vi "运维调试_总磷总氮.vi"() -> ()   [LabVIEW 2016, in "斯坦道氨氮.lvlib"]
uses:
  <vilib>/Utility/miscctls.llb/LVPointTypeDef.ctl
  <vilib>/Plasmionique/MB Master/MB_Master/MB_Master.lvclass
  <vilib>/ptbypt/NI_PtbyPt.lvlib
panel:
  out "步骤":u16
  out "seconds since 1Jan1904 2":timestamp
  out "seconds since 1Jan1904":timestamp
  in  "周期设置":bool
  in  "流程操作":bool
  out "消解压力":sgl format="%#.2f kPa"
  out "权限等级":string
  out "总步数":i32
  out "滑动杆":dbl(slide) caption="测试进度" scale=0.0..100.0
  out "试剂余量显示":sgl[][](graph)
  in  "仪器校准":bool
  in  "参数查询":bool
  out "简易步骤名称":string
  in  "温度曲线":bool
  in  "试剂余量":bool
  in  "灯值调整":bool
  out "固件版本号":string
  out "模块版本号":string
  out "注射器温度":sgl format="%#.2f ℃"
  out "消解温度":sgl format="%#.2f ℃"
  out "ADC":sgl
  out "F3":sgl format="%#.6f"
  out "F2":sgl format="%#.6f"
  out "F1":sgl format="%#.6f"
  out "F0":sgl format="%#.6f"
  out "运行状态":T1 {"数据时间:" format="%<%y/%m/%d %H:%M:%S>T"; "仪器时间:" format="%<%y/%m/%d %H:%M:%S>T"}
  in  "单选按钮":T2=enum."总氮"
  in  "布尔":bool
  in  "外设固件":bool
  out "字符串 2":string
  in  "数组":string[](array[string])
  in  "返回":bool
  in  "参数设置":bool
  out "集成报警信息":string
  in  "停止":bool
  in  "手动启动":bool
  in  "调试":bool
  out "多列列表框":i32(listbox)
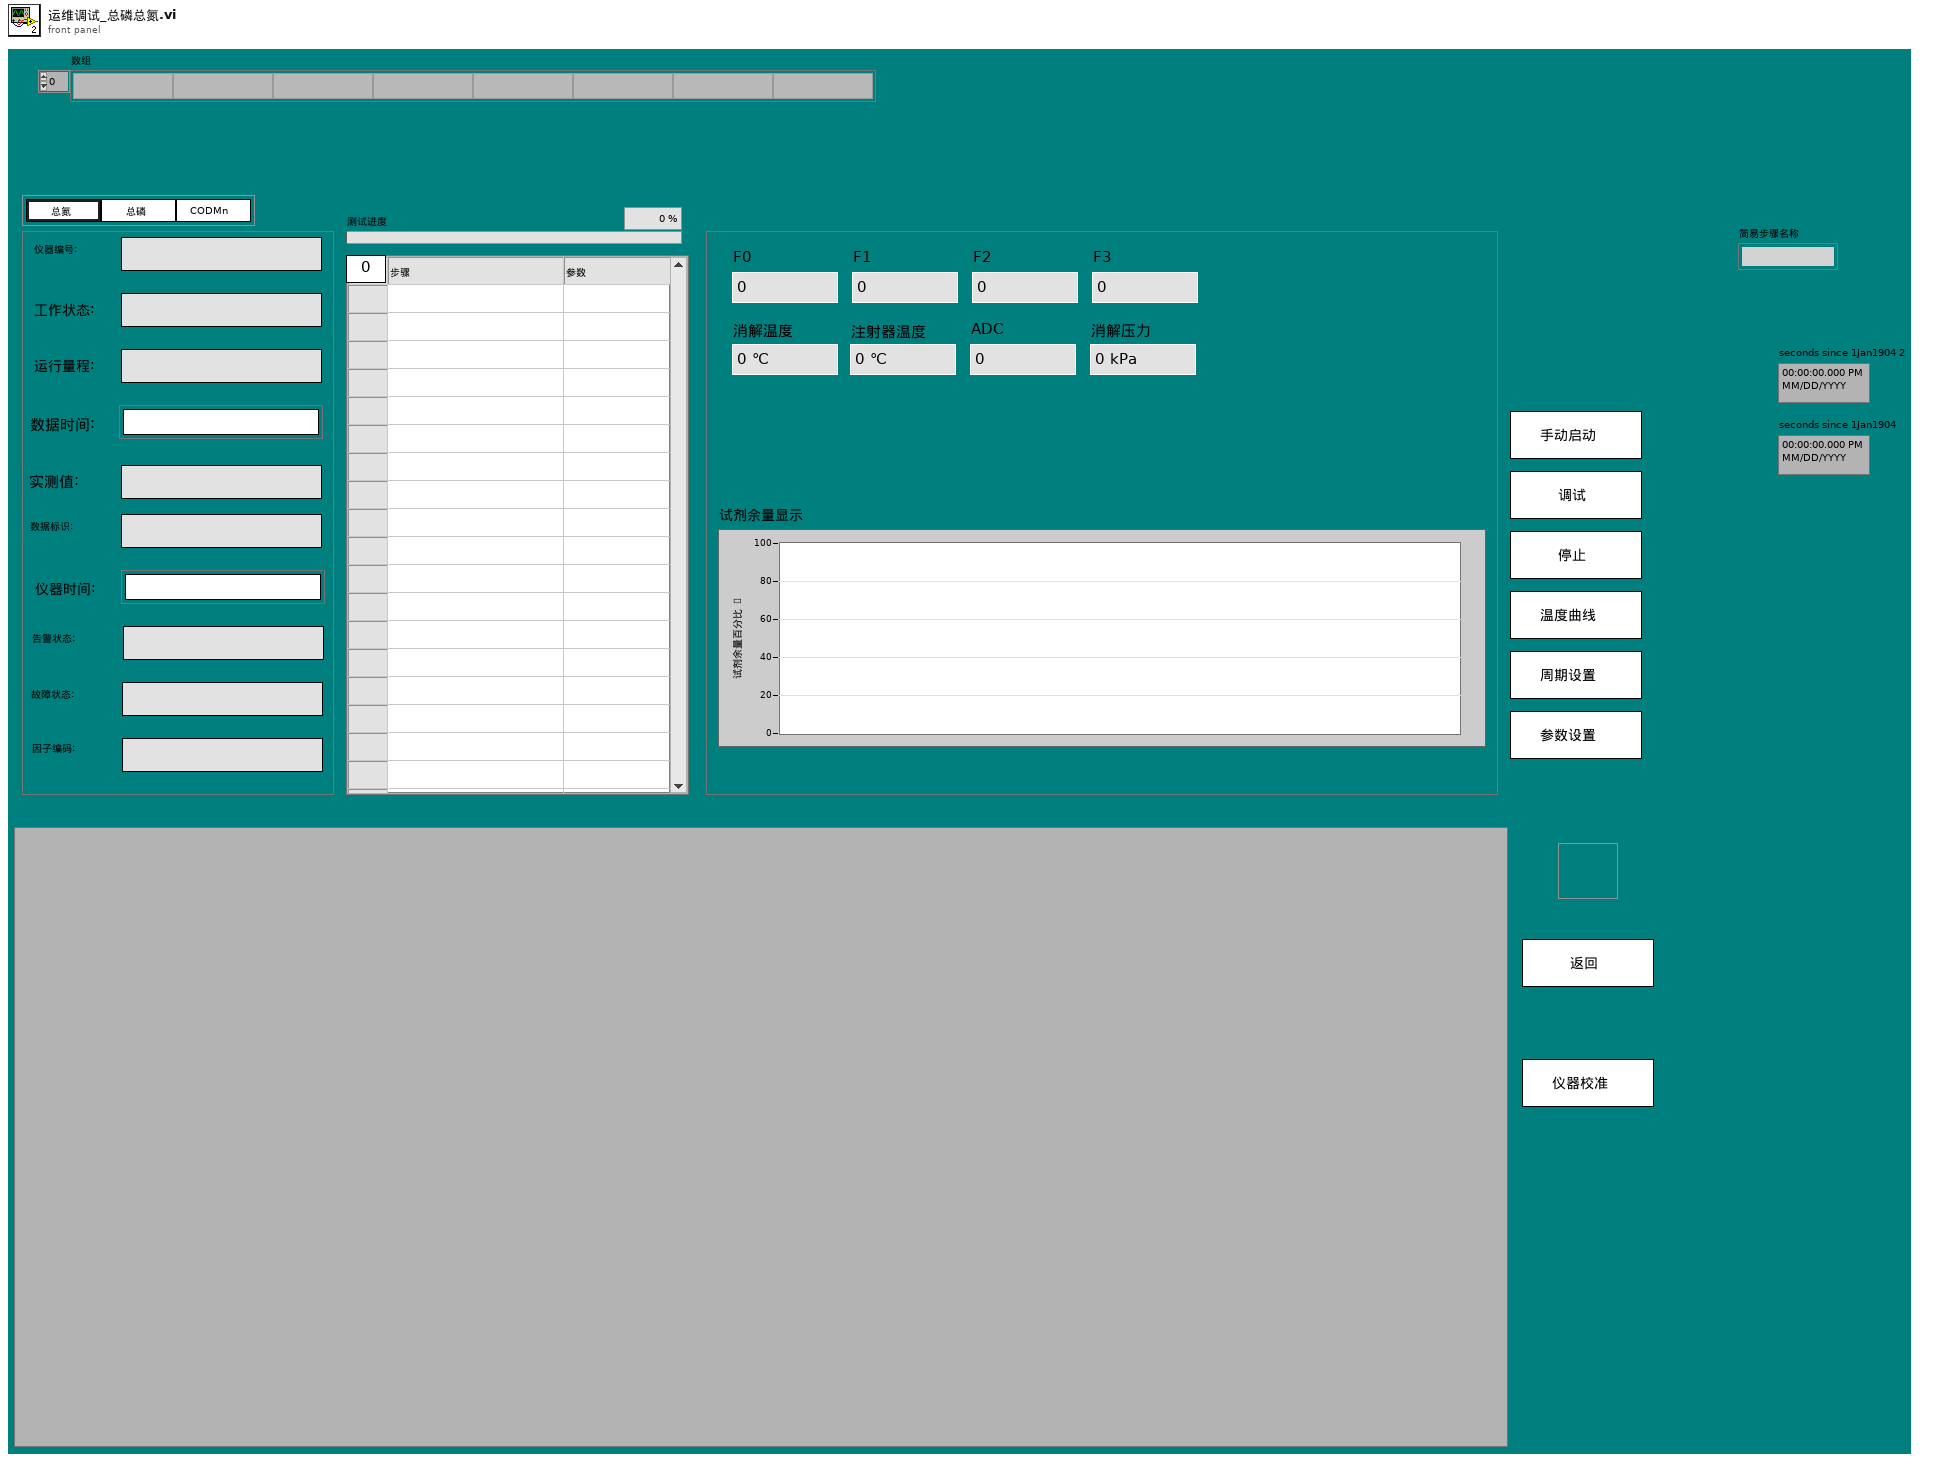
[diagram p1: front panel]
types:
  T1 = cluster{"仪器编号:":string, "工作状态:":string, "运行量程: ":string, "数据时间:":timestamp, "实测值:":string, "数据标识: ":string, "仪器时间:":timestamp, "告警状态: ":string, "故障状态:  ":string, "因子编码:":string}
  T2 = typedef "斯坦道氨氮.lvlib/启动参数显示控件.ctl" = enum32{"COD", "氨氮", "总氮", "总磷", "磷酸盐", "硝氮", "亚硝氮", "硅酸盐", "硫化物", "氟化物", "CODMn"}
  T3 = typedef "LVPointTypeDef.ctl" = cluster{"Horizontal":i16, "Vertical":i16}
  T4 = cluster{"系统时间":timestamp, "工作状态":u16, "测量模式":enum16{"待机", "连续模式", "周期模式", "定点模式", "受控模式", "手动模式"}, "告警代码":u16, "故障代码":u16, "日志代码":u16, "软件版本":u16, "F0":sgl, "F1":sgl, "F2":sgl, "F3":sgl, "T":sgl, "H":sgl, "id":u16, "flowid":u16, "量程":u16, "总磷控温温度1":sgl, "营养盐控温温度2":sgl, "ADC":sgl, "结果值":sgl, "运行时间":u16, "步骤详情":string, "步骤流程":string}
  T5 = typedef "报警信息字段定义.ctl" = cluster{"时间":timestamp, "参数":string, "元器件":string, "故障现象":string, "故障分析":string, "state":string, "code":string, "platform_alarm_code":string, "是否上报":string}
  T6 = typedef "Alarm interface.lvlib/报警短信语音交互.ctl" = cluster{"参数":string, "元器件":string, "故障现象":string, "code":string, "platform_alarm_code":string, "solutionList":cluster{"reason":string, "solution":string}[], "是否上报":string}
  T7 = cluster{"Major":u16, "Minor":u16, "Fix":u16, "Build":u16}
  T8 = typedef "LVStringsAndValuesArrayTypeDef_U16.ctl" = cluster{"String":string, "Value":u16}[]
  T9 = cluster{"因子编码":u32, "单位":u16, "标样参考值":sgl, "水样数据时间":timestamp, "水样实测值":sgl, "水样数据标识":string, "标样数据时间":timestamp, "标样实测值":sgl, "标样数据标识":string, "空白数据时间":timestamp, "空白实测值":sgl, "空白数据标识":string, "零点核查数据时间":timestamp, "零点核查实测值":sgl, "零点核查数据标识":string, "跨度核查数据时间":timestamp, "跨度核查实测值":sgl, "跨度核查数据标识":string, "加标回收数据时间":timestamp, "加标回收实测值":sgl, "加标回收数据标识":string, "平行样数据时间":timestamp, "平行样实测值":sgl, "平行样数据标识":string, "F0":sgl, "F1":sgl, "F2":sgl, "F3":sgl, "F4":sgl, "F5":sgl, "F6":sgl, "F7":sgl, "温度":sgl, "湿度":sgl, "X值":sgl, "fidrange":u16, "X1值":sgl}[]
  T10 = typedef "SingleStepTestV3.lvlib/SingleStepTestV3.lvclass/仪器版本.ctl" = enum16{"V3.1版", "V4版", "V3版", "V4.2版"}
  T11 = cluster{"因子编码":u32, "单位":u16, "标样参考值":sgl, "水样数据时间":timestamp, "水样实测值":sgl, "水样数据标识":string, "标样数据时间":timestamp, "标样实测值":sgl, "标样数据标识":string, "空白数据时间":timestamp, "空白实测值":sgl, "空白数据标识":string, "零点核查数据时间":timestamp, "零点核查实测值":sgl, "零点核查数据标识":string, "跨度核查数据时间":timestamp, "跨度核查实测值":sgl, "跨度核查数据标识":string, "加标回收数据时间":timestamp, "加标回收实测值":sgl, "加标回收数据标识":string, "平行样数据时间":timestamp, "平行样实测值":sgl, "平行样数据标识":string, "F0":sgl, "F1":sgl, "F2":sgl, "F3":sgl, "F4":sgl, "F5":sgl, "F6":sgl, "F7":sgl, "温度":sgl, "湿度":sgl, "X值":sgl, "fidrange":u16, "X1值":sgl}
  T12 = typedef "TimingControl.lvlib/TimingControl.lvclass/国标控制命令.ctl" = enum16{"启动测量", "标样核查", "零点核查", "跨度核查", "空白测试", "平行样测试", "加标回收", "空白校准", "标样校准", "初始化（清洗）", "停止测试", "仪器重启", "校时", "模式设置", "测量间隔设置"}
  T13 = typedef "TimingControl.lvlib/TimingControl.lvclass/测量参数.ctl" = u16
  T14 = enum32{"Bad", "Idle", "Run top level", "Running"}
  T15 = cluster{"时间标识":timestamp, "设备":string, "日志信息":string, "流程参数":string}
  T16 = typedef "LVRowAndColumnUnsignedTypeDef.ctl" = cluster{"Row":u32, "Column":u32}
  T17 = typedef "操作日志字段定义.ctl" = cluster{"时间":timestamp, "参数":string, "日志信息":string, "流程参数":string}
  T18 = cluster{"站号":u16, "量程切换":enum32{"H", "L", "AUTO"}, "控制命令":enum16{"启动测量", "标样核查", "零点核查", "跨度核查", "空白测试", "平行样测试", "加标回收", "空白校准", "标样校准", "初始化（清洗）", "停止测试", "仪器重启", "校时", "模式设置", "测量间隔设置"}, "模式设置":enum16{"待机", "连续模式", "周期模式", "定点模式", "受控模式", "手动模式"}, "测量间隔":u16}
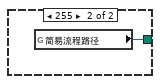
[diagram p6: hidden frame]
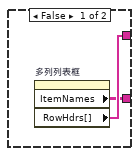
[diagram p7: hidden frame]
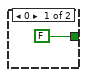
[diagram p11: hidden frame]
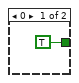
[diagram p18: hidden frame]
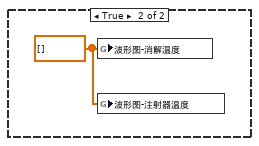
[diagram p19: hidden frame]
diagram:
  n1 = Obtain Queue(name (unnamed)="balloon" ("名称（未命名）"), element data type=cluster{"Title":string, "Body":string} {"Title"="", "Body"=""}) -> (queue out=w1:refnum<queue>)  [unwired: 3 in, 2 out]
  n2 = flat-sequence {
    frame #0 {
      n3 = property on="窗格" class="Pane"("Origin"=T3 {"Horizontal"=0, "Vertical"=0} ("原点")) -> ()  [unwired: 2 in, 2 out]
    }
  }
  n4 = while {
    stop <- FALSE stop-if-true
    n5 = global read "VAR总磷总氮全局变量.vi" "状态告警区"() -> (w32:T4)
    n6 = Wait (ms)(milliseconds to wait=u32 1000 ("等待时间（毫秒）")) -> ()  [unwired: 1 out]
    n7 = Unbundle By Name(w32) -> ("工作状态"=w30:u16)
    n8 = global read "VAR总磷总氮全局变量.vi" "通讯状态"() -> (w33:bool)
    n9 = Equal To 0?(x=w30) -> (x = 0?=w29:bool)
    n10 = And(x=w29, y=w33) -> (x .and. y?=w31:bool)
    n11 = call <vilib>:"Boolean Crossing PtByPt.vi"("input"=w31) -> ("crossing"=w28:bool)  [unwired: 2 in]
    n12 = case shown="True" w28 {
      frame False {
      }
      frame True {
        n13 = control-ref of="试剂余量显示"() -> (w36:refnum<vi>)
        n14 = call "试剂余量展示.vi"("波形图 2"=w36) -> ("波形图"=→"试剂余量显示":sgl[][])  [unwired: 10 in]
      }
    }
  }
  n15 = while {
    shift-right: [w39] -> _
    shift-left: _ -> [w41]
    tunnel: w1 -> [w38]
    stop <- FALSE stop-if-true
    n16 = global read "VAR总磷总氮全局变量.vi" "状态告警区"() -> (w47:T4)
    n17 = Wait (ms)(milliseconds to wait=u32 100 ("等待时间（毫秒）")) -> ()  [unwired: 1 out]
    n18 = Unbundle By Name(w47) -> ("工作状态"=w46:u16, "id"=w45:u16, "日志代码"=w44:u16, "故障代码"=w43:u16, "告警代码"=w42:u16)
    n19 = case shown="1, Default" w46 {
      tunnel: w45 -> [_ w51]
      tunnel: w44 -> [_ w54]
      tunnel: w43 -> [_ w53]
      tunnel: w42 -> [_ w52]
      tunnel: w41 -> [w49 w57]
      tunnel: [w49 w55] -> w39
      tunnel: w38 -> [_ w50]
      frame 0 {
      }
      frame 1, Default {
        n20 = Add(x=w53, y=w52) -> (x+y=w55:u16)
        n21 = Not Equal To 0?(x=w55) -> (x != 0?=w59:bool)
        n22 = Not Equal?(x=w55, y=w57) -> (x != y?=w58:bool)
        n23 = And(x=w59, y=w58) -> (x .and. y?=w56:bool)
        n24 = case shown="True" w56 {
          tunnel: w54 -> [_ _]
          tunnel: w53 -> [_ w64]
          tunnel: w52 -> [_ w63]
          tunnel: w51 -> [_ w60]
          tunnel: w50 -> [_ w68]
          frame False {
          }
          frame True {
            n25 = Not Equal To 0?(x=w64) -> (x != 0?=w66:bool)
            n26 = Not Equal To 0?(x=w63) -> (x != 0?=w62:bool)
            n27 = call "故障码字段定义.vi"("id"=w60, "故障代码"=w64) -> ("告警信息"=w65:T6)  [unwired: 9 in]
            n28 = call "告警码字段定义.vi"("id"=w60, "告警代码"=w63) -> ("告警信息"=w61:T6)  [unwired: 9 in]
            n29 = case shown="True" w66 {
              tunnel: w65 -> [_ w88]
              frame False {
              }
              frame True {
                n30 = Unbundle By Name(w88) -> ("参数"=w87:string, "元器件"=w86:string, "故障现象"=w85:string, "code"=w84:string, "platform_alarm_code"=w83:string, "是否上报"=w82:string)
                n31 = Get Date/Time In Seconds() -> (seconds since 1Jan1904=w89:timestamp)
                n32 = Bundle By Name(cluster=T5 {"时间"=timestamp(0 s since 1904-01-01), "参数"="", "元器件"="", "故障现象"="", "故障分析"="", "state"="", "code"="", "platform_alarm_code"="", "是否上报"=""} ("data in"), "时间"=w89, "参数"=w87, "元器件"=w86, "故障现象"=w85, "code"=w84, "platform_alarm_code"=w83, "是否上报"=w82) -> (w81:T5)
                n33 = call "总磷总氮报警信息.vi"("data in"=w81) -> ()  [unwired: 10 in, 1 out]
              }
            }
            n34 = Unbundle By Name(w65) -> ("故障现象"=w70:string)
            n35 = Unbundle By Name(w61) -> ("故障现象"=w69:string)
            n36 = case shown="True" w62 {
              tunnel: w61 -> [_ w71]
              frame False {
              }
              frame True {
                n37 = Unbundle By Name(w71) -> ("参数"=w75:string, "元器件"=w76:string, "故障现象"=w77:string, "code"=w78:string, "platform_alarm_code"=w79:string, "是否上报"=w80:string)
                n38 = Get Date/Time In Seconds() -> (seconds since 1Jan1904=w74:timestamp)
                n39 = Bundle By Name(cluster=T5 {"时间"=timestamp(0 s since 1904-01-01), "参数"="", "元器件"="", "故障现象"="", "故障分析"="", "state"="", "code"="", "platform_alarm_code"="", "是否上报"=""} ("data in"), "时间"=w74, "参数"=w75, "元器件"=w76, "故障现象"=w77, "code"=w78, "platform_alarm_code"=w79, "是否上报"=w80) -> (w72:T5)
                n40 = call "总磷总氮报警信息.vi"("data in"=w72) -> ()  [unwired: 10 in, 1 out]
              }
            }
            n41 = Bundle("故障现象"=w70, "故障现象"=w69) -> (w67:cluster{"故障现象":string, "故障现象":string})  [unwired: 1 in]
            n42 = Enqueue Element(queue=w68, element=w67) -> ()  [unwired: 2 in, 3 out]
          }
        }
      }
    }
  }
  n43 = flat-sequence {
    tunnel: [w137] -> w20
    tunnel: [errorcluster {"status"=FALSE, "code"=0, "source"=""} ("错误输入（无错误）")] -> w11
    tunnel: [errorcluster {"status"=FALSE, "code"=0, "source"=""} ("错误输入（无错误）")] -> w10
    tunnel: [w134] -> w8
    tunnel: [errorcluster {"status"=FALSE, "code"=0, "source"=""} ("error out")] -> w7
    tunnel: [errorcluster {"status"=FALSE, "code"=0, "source"=""} ("错误输入（无错误）")] -> w6
    frame #0 {
      n44 = global read "VAR总磷总氮全局变量.vi" "初始化"() -> (w91:bool)
      n45 = control-ref of="本VI"() -> (w99:refnum<vi>)
      n46 = case shown="False" w91 {
        frame False {
          n47 = call "配置初始化.vi"() -> ()  [unwired: 11 in, 1 out]
        }
        frame True {
        }
      }
      n48 = property class="VI"(reference=w99) -> ("Library.Version"=w98:T7)  [unwired: 1 in, 2 out]
      n49 = Unbundle By Name(w98) -> ("Major"=w96:u16, "Minor"=w95:u16, "Fix"=w94:u16, "Build"=w93:u16)
      n50 = Format Into String(format string="模块版本号：%d.%d.%d.%d" ("格式字符串"), w96, w95, w94, w93) -> (resulting string=→"模块版本号":string)  [unwired: 2 in, 1 out]
      n51 = call "新建通讯互斥锁.vi"() -> ()  [unwired: 11 in, 1 out]
    }
    frame #1 {
      n52 = vi-ref "斯坦道氨氮.lvlib:总磷总氮通讯.vi"() -> (w104:refnum<vi>)
      n53 = global read "model config var.vi" "启动队列名称"() -> (w102:cluster{"String":string, "Value":u16}[])
      n54 = vi-ref "斯坦道氨氮.lvlib:总磷总氮测量数据储存.vi"() -> (w112:refnum<vi>)
      n55 = property class="VI"(reference=w104) -> ("Name"=w105:string)  [unwired: 1 in, 2 out]
      n56 = Index Array(array=w102) -> (element=w101:cluster{"String":string, "Value":u16})  [unwired: 1 in]
      n57 = Unbundle By Name(w101) -> ("Value"=w100:u16)
      n58 = property class="VI"(reference=w112) -> ("Name"=w119:string)  [unwired: 1 in, 2 out]
      n59 = Open VI Reference(type specifier VI Refnum (for type only)=refnum<vi> refnum, vi path=w105, options=128 ("选项")) -> (vi reference=w107:refnum<vi>, error out=w109:errorcluster)  [unwired: 3 in]
      n60 = case shown="22" w100 {
        tunnel: [w120 启动参数显示控件."总磷" ("单选按钮") 启动参数显示控件."总氮" ("单选按钮") 启动参数显示控件."COD" ("单选按钮") 启动参数显示控件."氨氮" ("单选按钮") 启动参数显示控件."磷酸盐" ("单选按钮") 启动参数显示控件."硝氮" ("单选按钮") 启动参数显示控件."亚硝氮" ("单选按钮") 启动参数显示控件."硅酸盐" ("单选按钮") 启动参数显示控件."硫化物" ("单选按钮") 启动参数显示控件."氟化物" ("单选按钮") 启动参数显示控件."CODMn" ("单选按钮")] -> w103
        frame 0, Default {
          n61 = property on="单选按钮" class="RadioBtnsControl (strict)"() -> ("Value"=w120:T2)  [unwired: 2 in, 2 out]
        }
        frame 1 {
        }
        frame 2 {
        }
        frame 22 {
        }
        frame 3 {
        }
        frame 4 {
        }
        frame 5 {
        }
        frame 6 {
        }
        frame 7 {
        }
        frame 8 {
        }
        frame 50 {
        }
        frame 21 {
        }
      }
      n62 = call-by-ref "开始异步调用"(reference=w107, error in=w109) -> (reference out=w111:refnum<vi>, error out=w110:errorcluster)  [unwired: 12 in]
      n63 = Open VI Reference(type specifier VI Refnum (for type only)=refnum<vi> refnum, vi path=w119, options=128 ("选项")) -> (vi reference=w117:refnum<vi>, error out=w115:errorcluster)  [unwired: 3 in]
      n64 = Close Reference(reference=w111, error in (no error)=w110) -> ()  [unwired: 1 out]
      n65 = call-by-ref "开始异步调用"(reference=w117, error in=w115) -> (reference out=w113:refnum<vi>, error out=w114:errorcluster)  [unwired: 12 in]
      n66 = Close Reference(reference=w113, error in (no error)=w114) -> ()  [unwired: 1 out]
      n67 = property on="单选按钮" class="RadioBtnsControl (strict)"("Value"=w103) -> ()  [unwired: 2 in, 2 out]
    }
    frame #2 {
      n68 = call "配置文件路径.vi"() -> ("appended path"=w134:path)  [unwired: 11 in]
      n69 = call "设置模块队列名.vi"() -> ("Msg"=w137:string)  [unwired: 5 in]
    }
  }
  n70 = while {
    shift-right: [w147] -> _
    shift-left: u32 0 ("y") -> [w149]
    stop <- FALSE stop-if-true
    # "密码权限"
    n71 = global read "VAR总磷总氮全局变量.vi" "权限等级"() -> (w144:enum16{"一级权限", "二级权限", "三级权限", "超级权限"})
    n72 = case shown="False" "布尔" {
      tunnel: w149 -> [_ w162]
      tunnel: [_ w161] -> w147
      frame False {
      }
      frame True {
        n73 = Increment(x=w162) -> (x+1=w161:u32)
      }
    }
    n74 = Wait (ms)(milliseconds to wait=u32 1000 ("等待时间（毫秒）")) -> ()  [unwired: 1 out]
    n75 = case shown="\"超级权限\"" w144 {
      tunnel: [_ w154 w156 w159] -> w138
      tunnel: [_ _ w156 w159] -> _
      tunnel: [_ w154 w156 w159] -> w143
      tunnel: [_ _ _ TRUE] -> _
      tunnel: [TRUE _ _ _] -> w141
      tunnel: ["一级权限" "二级权限" "三级权限" "超级权限"] -> w139
      frame "一级权限", Default {
      }
      frame "二级权限" {
        w154 = TRUE
      }
      frame "三级权限" {
        w156 = TRUE
      }
      frame "超级权限" {
        w159 = TRUE
      }
    }
    "权限等级" <- w139
    n76 = property on="外设固件" class="Bool"("Visible"=w143) -> ()  [unwired: 2 in, 2 out]
    n77 = property on="流程操作" class="Bool"("Visible"=w138) -> ()  [unwired: 2 in, 2 out]
    n78 = property on="试剂余量" class="Bool"("Visible"=w138) -> ()  [unwired: 2 in, 2 out]
    n79 = property on="灯值调整" class="Bool"("Visible"=w138) -> ()  [unwired: 2 in, 2 out]
    n80 = Greater Or Equal?(x=w147, y=u32 3600) -> (x >= y?=w145:bool)
    n81 = Not(x=w141) -> (.not. x?=w140:bool)
    n82 = property on="布尔" class="Bool (strict)"("Value"=w140) -> ()  [unwired: 2 in, 2 out]
    n83 = case shown="True" w145 {
      frame False {
      }
      frame True {
        n84 = global write "VAR总磷总氮全局变量.vi" "权限等级"(enum16{"一级权限", "二级权限", "三级权限", "超级权限"}."一级权限" ("权限等级")) -> ()
      }
    }
  }
  n85 = while {
    shift-right: [w167] -> _
    shift-left: 0 -> [w168]
    stop <- FALSE stop-if-true
    n86 = global read "VAR总磷总氮全局变量.vi" "心跳包打开状态"() -> (w163:bool)
    n87 = Wait (ms)(milliseconds to wait=u32 1000 ("等待时间（毫秒）")) -> ()  [unwired: 1 out]
    n88 = case shown="False" w163 {
      tunnel: w168 -> [w172 _]
      tunnel: [w171 _] -> w167
      frame False {
        n89 = Increment(x=w172) -> (x+1=w171:i32)
      }
      frame True {
      }
    }
    n90 = Greater Or Equal?(x=w167, y=600) -> (x >= y?=w165:bool)
    n91 = case shown="True" w165 {
      frame False {
      }
      frame True {
        n92 = global write "VAR总磷总氮全局变量.vi" "升级固件关闭心跳包"(FALSE ("关闭心跳包")) -> ()
      }
    }
  }
  n93 = while {
    shift-right: [w174] -> _
    shift-left: TRUE -> [w175]
    stop <- FALSE stop-if-true
    n94 = global read "VAR总磷总氮全局变量.vi" "状态告警区"() -> (w178:T4)
    n95 = global read "VAR总磷总氮全局变量.vi" "状态告警区"() -> (w181:T4)
    n96 = Wait (ms)(milliseconds to wait=u32 1000 ("等待时间（毫秒）")) -> ()  [unwired: 1 out]
    n97 = Unbundle By Name(w181) -> ("工作状态"=w176:u16, "总磷控温温度1"=w180:sgl, "营养盐控温温度2"=w179:sgl)
    n98 = Unbundle By Name(w178) -> ("总磷控温温度1"=w177:sgl)
    n99 = call "消解压力计算.vi"("当前消解温度"=w177) -> ("消解压力"=→"消解压力":dbl)  [unwired: 10 in]
    n100 = case shown="1, Default" w176 {
      tunnel: w180 -> [_ w187]
      tunnel: w179 -> [_ w186]
      tunnel: w175 -> [_ w185]
      tunnel: [TRUE _] -> w174
      frame 0 {
      }
      frame 1, Default {
        n101 = case shown="False" w185 {
          tunnel: w187 -> [w193 _]
          tunnel: w186 -> [w192 _]
          frame False {
            n102 = global read "VAR总磷总氮全局变量.vi" "波形图-消解温度"() -> (w191:sgl[])
            n103 = global read "VAR总磷总氮全局变量.vi" "波形图-注射器温度"() -> (w190:sgl[])
            n104 = Build Array (concatenate)(w191, w193) -> (w189:sgl[])
            n105 = Build Array (concatenate)(w190, w192) -> (w188:sgl[])
            n106 = global write "VAR总磷总氮全局变量.vi" "波形图-消解温度"(w189) -> ()
            n107 = global write "VAR总磷总氮全局变量.vi" "波形图-注射器温度"(w188) -> ()
          }
          frame True {
            w194 = dbl[] [] ("波形图-消解温度")
            n108 = global write "VAR总磷总氮全局变量.vi" "波形图-消解温度"(w194) -> ()
            n109 = global write "VAR总磷总氮全局变量.vi" "波形图-注射器温度"(w194) -> ()
          }
        }
      }
    }
  }
  n110 = while {
    stop <- FALSE stop-if-true
    n111 = global read "VAR总磷总氮全局变量.vi" "状态告警区"() -> (w206:T4)
    n112 = Wait (ms)(milliseconds to wait=u32 1000 ("等待时间（毫秒）")) -> ()  [unwired: 1 out]
    n113 = Unbundle By Name(w206) -> ("id"=w205:u16, "flowid"=w204:u16, "量程"=w203:u16, "工作状态"=w196:u16)
    n114 = case shown="0, Default" w196 {
      tunnel: [w216 w217] -> w198
      frame 0, Default {
        n115 = global read "总磷总氮断电保存全局变量.vi" "流程路径"() -> (w216:path)
      }
      frame 255 {
        n116 = global read "总磷总氮断电保存全局变量.vi" "简易流程路径"() -> (w217:path)
      }
    }
    n117 = feedback #1() -> (w195:u16)  [unwired: 1 in]
    n118 = feedback-in #1(w196) -> ()
    n119 = Not Equal?(x=w195, y=w196) -> (x != y?=w212:bool)
    n120 = Not Equal To 0?(x=w196) -> (x != 0?=w207:bool)
    n121 = Bundle("id"=w205, "flowid"=w204, "量程"=w203) -> (w200:cluster{"id":u16, "flowid":u16, "量程":u16})  [unwired: 1 in]
    n122 = feedback #2() -> (w197:path)  [unwired: 1 in]
    n123 = feedback-in #2(w198) -> ()
    n124 = feedback-in #3(w200) -> ()
    n125 = feedback #3() -> (w201:cluster{"id":u16, "flowid":u16, "量程":u16})  [unwired: 1 in]
    n126 = Not Equal?(x=w197, y=w198) -> (x != y?=w211:bool)
    n127 = Not Equal?(x=w200, y=w201) -> (x != y?=w199:bool)
    n128 = Compound Arithmetic op=OR ("复合运算")(w211, w212, w199) -> (w213:bool)
    n129 = And(x=w207, y=w213) -> (x .and. y?=w208:bool)
    n130 = case shown="True" w208 {
      tunnel: [w219 w222] -> w210
      tunnel: [w218 w223] -> w214
      tunnel: w200 -> [_ w221]
      tunnel: w198 -> [_ w224]
      tunnel: w196 -> [_ w220]
      frame False {
        n131 = property on="多列列表框" class="MCListbox (strict)"() -> ("ItemNames"=w218:string[][], "RowHdrs[]"=w219:string[])  [unwired: 2 in, 2 out]
      }
      frame True {
        n132 = case shown="255" w220 {
          tunnel: w221 -> [_ w229]
          frame 0, Default {
          }
          frame 255 {
            n133 = Unbundle By Name(w229) -> ("id"=w228:u16, "flowid"=w226:u16)
            n134 = call "获取简易流程名称API.vi"("参数下拉列表"=w228) -> ("字符串与值[]"=w227:T8)  [unwired: 9 in, 1 out]
            n135 = for {
              tunnel: w227 -> [w234] mode=indexing
              tunnel: w226 -> [w232]
              tunnel: [w231] -> w225
              stop <- w230 stop-if-true
              n136 = Unbundle By Name(w234) -> ("String"=w231:string, "Value"=w233:u16)
              n137 = Equal?(x=w233, y=w232) -> (x = y?=w230:bool)
            }
            "简易步骤名称" <- w225
          }
        }
        n138 = call "斯坦道XML解析.vi"("工作状态"=w220, "添加的路径"=w224, "参数簇"=w221) -> ("步骤名"=w223:string[][], "索引"=w222:string[])  [unwired: 6 in, 1 out]
      }
    }
    n139 = Array Size(array=w210) -> (size(s)=→"总步数":i32)
    n140 = property on="多列列表框" class="MCListbox (strict)"("ItemNames"=w214, "RowHdrs[]"=w210) -> ()  [unwired: 2 in, 2 out]
  }
  n141 = while {
    shift-right: [w246] -> _
    shift-left: u16 1 ("工作状态") -> [w244]
    stop <- FALSE stop-if-true
    (unwired) "注射器温度"
    n142 = global write "VAR总磷总氮全局变量.vi" "最近一次工作状态"(w244) -> ()
    n143 = global read "VAR总磷总氮全局变量.vi" "状态告警区"() -> (w266:T4)
    n144 = global read "VAR总磷总氮全局变量.vi" "通讯状态"() -> (w277:bool)
    n145 = Wait (ms)(milliseconds to wait=u32 1000 ("等待时间（毫秒）")) -> ()  [unwired: 1 out]
    n146 = case shown="\"氨氮\"" "单选按钮" {
      tunnel: [22 3 2 1 4 5 6 7 8 50 21] -> w235
      tunnel: [_ TRUE _ _ _ _ _ _ _ _ _] -> w238
      frame "COD", Default {
      }
      frame "氨氮" {
      }
      frame "总氮" {
      }
      frame "总磷" {
      }
      frame "磷酸盐" {
      }
      frame "硝氮" {
      }
      frame "亚硝氮" {
      }
      frame "硅酸盐" {
      }
      frame "硫化物" {
      }
      frame "氟化物" {
      }
      frame "CODMn" {
      }
    }
    n147 = Unbundle By Name(w266) -> ("id"=w265:u16, "工作状态"=w261:u16)
    n148 = case shown="True" w277 {
      tunnel: ["通讯异常" ("集成报警信息") w396] -> w276
      frame False {
      }
      frame True {
        n149 = local read "seconds since 1Jan1904 2"() -> (w388:timestamp)
        n150 = local read "seconds since 1Jan1904"() -> (w391:timestamp)
        n151 = global read "VAR总磷总氮全局变量.vi" "状态告警区"() -> (w398:T4)
        n152 = Unbundle By Name(w398) -> ("工作状态"=w394:u16)
        n153 = Subtract(x=w388, y=w391) -> (x-y=w387:dbl)
        n154 = Not Equal To 0?(x=w394) -> (x != 0?=w390:bool)
        n155 = Get Date/Time In Seconds() -> (seconds since 1Jan1904=w389:timestamp)
        n156 = case shown="True" w390 {
          tunnel: w389 -> [_ w399]
          frame False {
          }
          frame True {
            "seconds since 1Jan1904 2" <- w399
          }
        }
        n157 = Greater Or Equal?(x=w387, y=36000.0) -> (x >= y?=w384:bool)
        n158 = call <vilib>:"Boolean Crossing PtByPt.vi"("direction"=enum16{"either", "false-true", "true-false"}."false-true", "input"=w390) -> ("crossing"=w392:bool)  [unwired: 1 in]
        n159 = Or(x=w392, y=w384) -> (x .or. y?=w385:bool)
        n160 = case shown="True" w385 {
          tunnel: w389 -> [_ w400]
          frame False {
          }
          frame True {
            "seconds since 1Jan1904" <- w400
          }
        }
        n161 = global read "VAR总磷总氮全局变量.vi" "测量状态"() -> (w395:string)
        n162 = Format Into String(format string="工作计时: %d 秒" ("格式字符串"), initial string=w395, w387) -> (resulting string=w396:string)  [unwired: 1 in, 1 out]
      }
    }
    "集成报警信息" <- w276
    n163 = global read "VAR总磷总氮全局变量.vi" "测量数据区数组"() -> (w250:T9)
    n164 = case shown="1, Default" w261 {
      tunnel: w265 -> [_ w333]
      frame 0 {
      }
      frame 1, Default {
        n165 = case shown="3" w333 {
          tunnel: [w334 启动参数显示控件."总磷" ("单选按钮") 启动参数显示控件."总氮" ("单选按钮") 启动参数显示控件."COD" ("单选按钮") 启动参数显示控件."氨氮" ("单选按钮") 启动参数显示控件."磷酸盐" ("单选按钮") 启动参数显示控件."硝氮" ("单选按钮") 启动参数显示控件."亚硝氮" ("单选按钮") 启动参数显示控件."硅酸盐" ("单选按钮") 启动参数显示控件."硫化物" ("单选按钮") 启动参数显示控件."CODMn" ("单选按钮") 启动参数显示控件."氟化物" ("单选按钮")] -> w332
          frame 0, Default {
            n166 = property on="单选按钮" class="RadioBtnsControl (strict)"() -> ("Value"=w334:T2)  [unwired: 2 in, 2 out]
          }
          frame 1 {
          }
          frame 2 {
          }
          frame 22 {
          }
          frame 3 {
          }
          frame 4 {
          }
          frame 5 {
          }
          frame 6 {
          }
          frame 7 {
          }
          frame 8 {
          }
          frame 21 {
          }
          frame 50 {
          }
        }
        n167 = property on="单选按钮" class="RadioBtnsControl (strict)"("Value"=w332) -> ()  [unwired: 2 in, 2 out]
      }
    }
    n168 = call "版本判断.vi"() -> ("仪器版本"=w240:T10)  [unwired: 11 in]
    n169 = call "id参数转换.vi"("id"=w235) -> ("数组资源索引"=w247:i32)  [unwired: 9 in, 1 out]
    n170 = case shown="\"V4版\", \"V4.2版\"" w240 {
      tunnel: [w280 "传感器" ("标题.文本")] -> w237
      tunnel: ["%#.2f ℃" ("数值文本.格式字符串") "%#.2f " ("数值文本.格式字符串")] -> w239
      tunnel: w238 -> [w283 _]
      frame "V3.1版", Default {
        n171 = Select(t="显色温度", s=w283, f="注射器温度" ("标题.文本")) -> (s? t:f=w280:string)
      }
      frame "V4版", "V4.2版" {
      }
    }
    n172 = Index Array(array=w250, index=w247) -> (element=w249:T11)
    n173 = case shown="0, Default" w244 {
      tunnel: [w301 w307 w311 w315 w319 w323 w327 w331] -> w260
      tunnel: [w299 w306 w310 w314 w317 w322 w326 w330] -> w255
      tunnel: [w302 w305 w309 w313 w316 w321 w325 w329] -> w253
      tunnel: w249 -> [_ w304 w308 w312 w318 w320 w324 w328]
      frame 0, Default {
        n174 = local read "运行状态"() -> (w303:T1)
        n175 = Unbundle By Name(w303) -> ("数据时间:"=w301:timestamp, "实测值:"=w300:string, "数据标识:"=w302:string)
        n176 = Fract/Exp String To Number(string=w300) -> (number=w299:dbl)  [unwired: 3 in, 1 out]
      }
      frame 1 {
        n177 = Unbundle By Name(w304) -> ("水样数据时间"=w307:timestamp, "水样实测值"=w306:sgl, "水样数据标识"=w305:string)
      }
      frame 2, 9 {
        n178 = Unbundle By Name(w308) -> ("标样数据时间"=w311:timestamp, "标样实测值"=w310:sgl, "标样数据标识"=w309:string)
      }
      frame 3 {
        n179 = Unbundle By Name(w312) -> ("零点核查数据时间"=w315:timestamp, "零点核查实测值"=w314:sgl, "零点核查数据标识"=w313:string)
      }
      frame 4 {
        n180 = Unbundle By Name(w318) -> ("跨度核查数据时间"=w319:timestamp, "跨度核查实测值"=w317:sgl, "跨度核查数据标识"=w316:string)
      }
      frame 7 {
        n181 = Unbundle By Name(w320) -> ("加标回收数据时间"=w323:timestamp, "加标回收实测值"=w322:sgl, "加标回收数据标识"=w321:string)
      }
      frame 5, 8 {
        n182 = Unbundle By Name(w324) -> ("空白数据时间"=w327:timestamp, "空白实测值"=w326:sgl, "空白数据标识"=w325:string)
      }
      frame 6 {
        n183 = Unbundle By Name(w328) -> ("平行样数据时间"=w331:timestamp, "平行样实测值"=w330:sgl, "平行样数据标识"=w329:string)
      }
    }
    n184 = Unbundle By Name(w249) -> ("因子编码"=w251:u32)
    n185 = global read "VAR总磷总氮全局变量.vi" "状态告警区"() -> (w275:T4)
    n186 = Unbundle By Name(w275) -> ("flowid"=w243:u16, "系统时间"=w271:timestamp, "工作状态"=w270:u16, "告警代码"=w264:u16, "故障代码"=w263:u16, "量程"=w269:u16)
    n187 = case shown="2" w270 {
      selector: w270 -> [w350 _ w356 w360 w363 w365 w367 w369 w371 w373 w375 w377 w379 w382]
      tunnel: [w351 "空闲" ("工作状态") "水样测量" ("工作状态") w359 "零点核查" ("工作状态") "跨度核查" ("工作状态") "空白测试" ("工作状态") "平行样测试" ("工作状态") "加标回收" ("工作状态") "空白校准" ("工作状态") "标样校准" ("工作状态") "初始化" ("工作状态") "单步调试" ("工作状态") w381] -> w245
      tunnel: [w349 w354 w356 w360 w363 w365 w367 w369 w371 w373 w375 w377 w379 w382] -> w246
      tunnel: w244 -> [w349 w354 _ _ _ _ _ _ _ _ _ _ _ _]
      tunnel: w243 -> [_ _ _ w358 _ _ _ _ _ _ _ _ _ _]
      frame Default {
        n188 = Format Into String(format string="%d" ("格式字符串"), initial string="未知" ("工作状态"), w350) -> (resulting string=w351:string)  [unwired: 1 in, 1 out]
      }
      frame 0 {
      }
      frame 1 {
      }
      frame 2 {
        n189 = case shown="5" w358 {
          tunnel: ["标样核查" ("工作状态") "快捷测试" ("工作状态")] -> w359
          frame 0, Default {
          }
          frame 5 {
          }
        }
      }
      frame 3 {
      }
      frame 4 {
      }
      frame 5 {
      }
      frame 6 {
      }
      frame 7 {
      }
      frame 8 {
      }
      frame 9 {
      }
      frame 10 {
      }
      frame 254 {
      }
      frame 255 {
        n190 = local read "简易步骤名称"() -> (w381:string)
      }
    }
    n191 = call "告警码字段定义.vi"("id"=w235, "告警代码"=w264) -> ("告警信息"=w242:T6)  [unwired: 9 in]
    n192 = call "故障码字段定义.vi"("id"=w235, "故障代码"=w263) -> ("告警信息"=w262:T6)  [unwired: 9 in]
    n193 = Unbundle By Name(w242) -> ("故障现象"=w241:string)
    n194 = Unbundle By Name(w262) -> ("故障现象"=w236:string)
    n195 = property on="注射器温度" class="DigNum (strict)"("Caption.Text"=w237, "NumText.FormatString"=w239) -> ()  [unwired: 2 in, 2 out]
    n196 = case shown="1" w269 {
      tunnel: ["" ("字符串") "低量程 " ("字符串") "高量程 " ("字符串")] -> w268
      frame Default {
      }
      frame 0 {
      }
      frame 1 {
      }
    }
    n197 = Number To Fractional String(number=w255, precision (6)=i16 4 ("精度(6)")) -> (F-format string=w257:string)  [unwired: 2 in]
    n198 = Concatenate Strings(w257, " " ("字符串"), "mg/L" ("字符串")) -> (w254:string)
    n199 = global read "VAR总磷总氮全局变量.vi" "序列号"() -> (w272:string)
    n200 = Format Into String(format string="w%05d" ("格式字符串"), w251) -> (resulting string=w267:string)  [unwired: 2 in, 1 out]
    n201 = global write "VAR总磷总氮全局变量.vi" "工作状态:"(w245) -> ()
    n202 = Bundle By Name(cluster=T1 {"仪器编号:"="", "工作状态:"="", "运行量程: "="", "数据时间:"=timestamp(0 s since 1904-01-01), "实测值:"="", "数据标识: "="", "仪器时间:"=timestamp(0 s since 1904-01-01), "告警状态: "="", "故障状态:  "="", "因子编码:"=""} ("运行状态"), "仪器编号:"=w272, "仪器时间:"=w271, "工作状态:"=w245, "告警状态:"=w241, "故障状态:"=w236, "运行量程:"=w268, "数据时间:"=w260, "实测值:"=w254, "数据标识:"=w253, "因子编码:"=w267) -> (→"运行状态":T1)
  }
  n203 = while {
    shift-right: [w401] -> _
    shift-left: _ -> [w406]
    tunnel: w8 -> [w404]
    stop <- FALSE stop-if-true
    n204 = File/Directory Info(path=w404) -> (last mod=w401:timestamp, error out=w402:errorcluster)  [unwired: 1 in, 5 out]
    n205 = Wait (ms)(milliseconds to wait=u32 1000 ("等待时间（毫秒）")) -> ()  [unwired: 1 out]
    n206 = Not Equal?(x=w406, y=w401) -> (x != y?=w405:bool)
    n207 = case shown="True" w405 {
      tunnel: [_ w408] -> _
      tunnel: w402 -> [_ _]
      frame False {
      }
      frame True {
        n208 = call "配置初始化.vi"() -> ("error out"=w408:errorcluster)  [unwired: 11 in]
      }
    }
  }
  n209 = flat-sequence {
    tunnel: w7 -> [_]
    frame #0 {
      (unwired) u32 0 ("等待时间（毫秒）")
      n210 = control-ref of="周期设置"() -> (w413:refnum<vi>)
      n211 = call "试剂余量后台任务.vi"() -> ()  [unwired: 12 in]
      n212 = call "New TimingControl.vi"("Reference"=w413) -> ("error out"=w411:errorcluster, "TimingControl out"=w412:refnum<class "TimingControl.lvclass">)  [unwired: 9 in]
      n213 = call "taskqueue ref.vi"() -> ("队列输出"=w414:refnum<queue>)  [unwired: 10 in, 1 out]
      n214 = while {
        tunnel: w414 -> [w433]
        shift-right: [w426] -> w410
        shift-left: w412 -> [w431]
        shift-right: [w425] -> w409
        shift-left: w411 -> [w430]
        stop <- FALSE stop-if-true
        n215 = global read "VAR总磷总氮全局变量.vi" "状态告警区"() -> (w434:T4)
        n216 = Wait (ms)(milliseconds to wait=u32 500 ("等待时间（毫秒）")) -> ()  [unwired: 1 out]
        n217 = global read "model config var.vi" "启动队列名称"() -> (w420:cluster{"String":string, "Value":u16}[])
        n218 = Unbundle By Name(w434) -> ("工作状态"=w432:u16, "系统时间"=w428:timestamp)
        n219 = for {
          tunnel: w420 -> [w445] mode=indexing
          tunnel: [w444] -> w419 mode=indexing
          n220 = Unbundle By Name(w445) -> ("String"=w444:string)
        }
        n221 = case shown="1, Default" w432 {
          tunnel: [FALSE TRUE] -> w427
          frame 0 {
          }
          frame 1, Default {
          }
        }
        n222 = property class="TimingControl"(reference=w431, error in=w430, "Properties:仪器时间"=w428, "Properties:仪器运行状态"=w427) -> (reference out=w426:refnum<class "TimingControl.lvclass">, error out=w425:errorcluster, "Properties:命令输出"=w429:cluster{"启动":bool, "控制命令":T12, "测量参数":T13})
        n223 = Array To Spreadsheet String(delimiter (Tab)="/" ("分隔符(Tab)"), array=w419, 3:"" ("格式字符串")) -> (spreadsheet string=w422:string)
        n224 = Unbundle By Name(w429) -> ("启动"=w416:bool, "控制命令"=w418:T12)
        n225 = Insert Into Array(array=w419, new element=w422) -> (w421:string[])  [unwired: 1 in]
        n226 = Bundle(w421) -> ()  [unwired: 1 in, 1 out]
        n227 = Bundle("控制命令"=w418, "") -> (w417:cluster{"控制命令":T12, string})  [unwired: 1 in]
        n228 = case shown="True" w416 {
          tunnel: w417 -> [_ w438]
          tunnel: w433 -> [_ w441]
          frame False {
          }
          frame True {
            n229 = Get Queue Status(queue=w441) -> (queue out=w439:refnum<queue>, # elements in queue=w440:i32)  [unwired: 2 in, 6 out]
            n230 = Equal To 0?(x=w440) -> (x = 0?=w437:bool)
            n231 = case shown="True" w437 {
              tunnel: w439 -> [_ w443]
              tunnel: w438 -> [_ w442]
              frame False {
              }
              frame True {
                n232 = Enqueue Element(queue=w443, element=w442) -> ()  [unwired: 2 in, 3 out]
              }
            }
          }
        }
      }
      n233 = call "task.vi"() -> ()  [unwired: 12 in]
      n234 = call "Close TimingControl.vi"("error in (no error)"=w409, "TimingControl in"=w410) -> ()  [unwired: 9 in, 1 out]
    }
  }
  n235 = while {
    tunnel: w7 -> [_]
    stop <- FALSE stop-if-true
    n236 = flat-sequence {
      frame #0 {
        n237 = global read "model config var.vi" "启动队列名称"() -> (w449:cluster{"String":string, "Value":u16}[])
        n238 = for {
          tunnel: w449 -> [w457] mode=indexing
          shift-right: [w456] -> w452
          shift-left: "" -> [w455]
          tunnel: [w454] -> w450 mode=indexing
          n239 = Unbundle By Name(w457) -> ("String"=w454:string)
          n240 = Concatenate Strings(w455, w454) -> (w456:string)
        }
        n241 = property on="单选按钮" class="RadioBtnsControl (strict)"() -> ("Controls[]"=w451:refnum<vi>[])  [unwired: 2 in, 2 out]
        n242 = global write "VAR总磷总氮全局变量.vi" "模块名称"(w452) -> ()
        n243 = for {
          tunnel: w451 -> [w465] mode=indexing
          tunnel: w450 -> [w464]
          n244 = property class="Ctl"(reference=w465) -> (reference out=w463:refnum<vi>, "Label.Text"=w459:string)  [unwired: 1 in, 1 out]
          n245 = case shown="\"COD\"" w459 {
            selector: w459 -> [w466 _]
            tunnel: [w466 "CODcr"] -> w458
            frame Default {
            }
            frame "COD" {
            }
          }
          n246 = Search 1D Array(1D array=w464, element=w458) -> (index of element=w462:i32)  [unwired: 1 in]
          n247 = Not Equal?(x=w462, y=-1) -> (x != y?=w460:bool)
          n248 = property class="Ctl"(reference=w463, "Visible"=w460) -> ()  [unwired: 1 in, 2 out]
        }
      }
      frame #1 {
        n249 = Wait (ms)(milliseconds to wait=u32 1000 ("等待时间（毫秒）")) -> ()  [unwired: 1 out]
      }
    }
  }
  n250 = call "时间延迟"("error in (no error)"=w6) -> ("error out"=w26:errorcluster)  [unwired: 10 in]
  n251 = vi-ref "斯坦道氨氮.lvlib:校准设置页.vi"() -> (w15:refnum<vi>)
  n252 = vi-ref "斯坦道氨氮.lvlib:参数设置页.vi"() -> (w19:refnum<vi>)
  n253 = property class="VI"(reference=w15, error in=w10) -> (reference out=w13:refnum<vi>, "Exec.State"=w14:T14)  [unwired: 1 out]
  n254 = property class="VI"(reference=w19, error in=w11) -> (reference out=w17:refnum<vi>, "Exec.State"=w18:T14)  [unwired: 1 out]
  n255 = while {
    tunnel: w26 -> [_]
    stop <- FALSE stop-if-true
    n256 = Wait (ms)(milliseconds to wait=u32 1000 ("等待时间（毫秒）")) -> ()  [unwired: 1 out]
    n257 = global read "VAR总磷总氮全局变量.vi" "状态告警区"() -> (w494:T4)
    n258 = global read "VAR总磷总氮全局变量.vi" "状态告警区"() -> (w495:T4)
    n259 = global read "VAR总磷总氮全局变量.vi" "状态告警区"() -> (w493:T4)
    n260 = global read "VAR总磷总氮全局变量.vi" "状态告警区"() -> (w491:T4)
    n261 = Unbundle By Name(w495) -> ("F0"=→"F0":sgl, "F1"=→"F1":sgl, "F2"=→"F2":sgl, "F3"=→"F3":sgl, "ADC"=→"ADC":sgl, "总磷控温温度1"=→"消解温度":sgl, "营养盐控温温度2"=→"注射器温度":sgl)
    n262 = Unbundle By Name(w494) -> ("日志代码"=w469:u16)
    "步骤" <- w469
    n263 = Unbundle By Name(w491) -> ("日志代码"=w490:u16)
    n264 = Unbundle By Name(w493) -> ("flowid"=w473:u16, "工作状态"=w486:u16, "id"=w487:u16)
    n265 = case shown="0" w486 {
      frame 0 {
        n266 = local write "数组"(string[] [] ("数组")) -> ()
      }
      frame 1, Default {
      }
    }
    n267 = feedback #4() -> (w492:u16)  [unwired: 1 in]
    n268 = feedback-in #4(w490) -> ()
    n269 = Not Equal To 0?(x=w486) -> (x != 0?=w471:bool)
    n270 = property on="总步数" class="DigNum (strict)"() -> ("Value"=w476:i32)  [unwired: 2 in, 2 out]
    n271 = Divide(x=w469, y=w476) -> (x/y=w475:dbl)
    n272 = Not Equal?(x=w490, y=w492) -> (x != y?=w489:bool)
    n273 = call <vilib>:"Boolean Crossing PtByPt.vi"("direction"=enum16{"either", "false-true", "true-false"}."either", "input"=w471) -> ("crossing"=w484:bool)  [unwired: 1 in]
    n274 = feedback-in #5(w469) -> ()
    n275 = feedback #5() -> (w497:u16)  [unwired: 1 in]
    n276 = Subtract(x=w469, y=1) -> (x-y=→"多列列表框":i32)
    n277 = case shown="True" w484 {
      tunnel: w487 -> [_ w520]
      tunnel: w473 -> [_ w508]
      tunnel: w471 -> [_ w506]
      frame False {
      }
      frame True {
        n278 = global read "VAR总磷总氮全局变量.vi" "最近一次工作状态"() -> (w507:u16)
        n279 = case shown="1" w507 {
          selector: w507 -> [w526 _ _ _ _ _ _ _ _ _ _ _]
          tunnel: [w525 "【水样测试】" ("字符串") w529 "【零点核查】" ("字符串") "【跨度核查】" ("字符串") "【空白测试】" ("字符串") "【平行样测试】" ("字符串") "【加标回收】" ("字符串") "【空白校准】" ("字符串") "【标样校准】" ("字符串") "【单步调试】" ("字符串") "【简易流程】" ("字符串")] -> w501
          tunnel: w508 -> [_ _ w528 _ _ _ _ _ _ _ _ _]
          frame 0, Default {
            n280 = Number To Decimal String(number=w526) -> (decimal integer string=w525:string)  [unwired: 1 in]
          }
          frame 1 {
          }
          frame 2 {
            n281 = case shown="0, Default" w528 {
              tunnel: ["【标样核查】" ("字符串") "【快捷测试】" ("字符串")] -> w529
              frame 0, Default {
              }
              frame 5 {
              }
            }
          }
          frame 3 {
          }
          frame 4 {
          }
          frame 5 {
          }
          frame 6 {
          }
          frame 7 {
          }
          frame 8 {
          }
          frame 9 {
          }
          frame 254 {
          }
          frame 255 {
          }
        }
        n282 = global read "VAR总磷总氮全局变量.vi" "状态告警区"() -> (w518:T4)
        n283 = Concatenate Strings("<<" ("字符串"), w501, "启动" ("字符串")) -> (w500:string)
        n284 = Unbundle By Name(w518) -> ("F0"=w517:sgl, "F1"=w516:sgl, "F2"=w515:sgl, "F3"=w514:sgl, "id"=w513:u16, "flowid"=w512:u16, "量程"=w511:u16)
        n285 = Concatenate Strings(w501, "停止>>" ("字符串")) -> (w504:string)
        n286 = Format Into String(format string="F0=%#f,F1=%#f,F2=%#f,F3=%#f,Flow=%d-%-d-%-d" ("格式字符串"), w517, w516, w515, w514, w513, w512, w511) -> (resulting string=w509:string)  [unwired: 2 in, 1 out]
        n287 = Select(t=w500, s=w506, f=w504) -> (s? t:f=w505:string)
        n288 = call "id参数转换.vi"("id"=w520) -> ("table输出"=w519:string)  [unwired: 9 in, 1 out]
        n289 = Get Date/Time In Seconds() -> (seconds since 1Jan1904=w523:timestamp)
        n290 = Bundle By Name(cluster=T15 {"时间标识"=timestamp(0 s since 1904-01-01), "设备"="", "日志信息"="", "流程参数"=""} ("data in"), "时间标识"=w523, "设备"=w519, "日志信息"=w505, "流程参数"=w509) -> (w522:T15)
        n291 = call "总磷总氮操作日志.vi"("data in"=w522) -> ()  [unwired: 10 in, 1 out]
      }
    }
    n292 = case shown="True" w489 {
      frame False {
      }
      frame True {
        n293 = property on="多列列表框" class="MCListbox (strict)"() -> ("ItemNames"=w546:string[][], "Value"=w542:i32)  [unwired: 2 in, 2 out]
        n294 = Index Array(array=w546, index (row)=w542) -> (element=w545:string[])  [unwired: 1 in]
        n295 = Index Array(array=w545) -> (element=w544:string)  [unwired: 1 in]
        n296 = call "过滤筛选流程.vi"("字符串"=w544) -> ("匹配后偏移量"=w543:i32)  [unwired: 10 in]
        n297 = case shown="Default" w543 {
          tunnel: w544 -> [w548 _]
          tunnel: w542 -> [w547 _]
          frame Default {
            n298 = case shown="\"读数\"" w548 {
              selector: w548 -> [w554 w561]
              tunnel: [w554 w561] -> w550
              tunnel: [string[] [] ("数组") w556] -> w549
              tunnel: w547 -> [_ w560]
              frame "读数" {
              }
              frame Default {
                n299 = Equal?(x=w560, y=1) -> (x = y?=w558:bool)
                n300 = Select(t=string[] [], s=w558, f="数组") -> (s? t:f=w556:string[])
              }
            }
            n301 = for {
              N: 1 -> [_]
              tunnel: w550 -> [w563]
              shift-right: [w562] -> w551
              shift-left: w549 -> [w564]
              n302 = Search 1D Array(1D array=w564, element=w563) -> (index of element=w567:i32)  [unwired: 1 in]
              n303 = Format Into String(format string="%s" ("格式字符串"), w563) -> (resulting string=w568:string)  [unwired: 2 in, 1 out]
              n304 = Equal?(x=w567, y=-1) -> (x = y?=w565:bool)
              n305 = case shown="True" w565 {
                tunnel: w568 -> [_ w578]
                tunnel: w564 -> [w570 w582]
                tunnel: w563 -> [_ w581]
                tunnel: [w570 w580] -> w562
                frame False {
                }
                frame True {
                  n306 = Insert Into Array(array=w582, new element=w581) -> (w580:string[])  [unwired: 1 in]
                  n307 = global read "VAR总磷总氮全局变量.vi" "状态告警区"() -> (w577:T4)
                  n308 = Unbundle By Name(w577) -> ("工作状态"=w576:u16, "flowid"=w571:u16)
                  n309 = case shown="2" w576 {
                    selector: w576 -> [w597 _ _ _ _ _ _ _ _ _ _ _]
                    tunnel: [w596 "【水样测试】" ("字符串") w600 "【零点核查】" ("字符串") "【跨度核查】" ("字符串") "【空白测试】" ("字符串") "【平行样测试】" ("字符串") "【加标回收】" ("字符串") "【空白校准】" ("字符串") "【标样校准】" ("字符串") "【单步调试】" ("字符串") w611] -> w574
                    tunnel: w571 -> [_ _ w599 _ _ _ _ _ _ _ _ _]
                    frame 0, Default {
                      n310 = Number To Decimal String(number=w597) -> (decimal integer string=w596:string)  [unwired: 1 in]
                    }
                    frame 1 {
                    }
                    frame 2 {
                      n311 = case shown="5" w599 {
                        tunnel: ["【标样核查】" ("字符串") "【快捷测试】" ("字符串")] -> w600
                        frame Default {
                        }
                        frame 5 {
                        }
                      }
                    }
                    frame 3 {
                    }
                    frame 4 {
                    }
                    frame 5 {
                    }
                    frame 6 {
                    }
                    frame 7 {
                    }
                    frame 8 {
                    }
                    frame 9 {
                    }
                    frame 254 {
                    }
                    frame 255 {
                      n312 = local read "简易步骤名称"() -> (w613:string)
                      n313 = Format Into String(format string="(%s)" ("格式字符串"), initial string="【简易流程】" ("工作状态"), w613) -> (resulting string=w611:string)  [unwired: 1 in, 1 out]
                    }
                  }
                  n314 = global read "VAR总磷总氮全局变量.vi" "状态告警区"() -> (w595:T4)
                  n315 = global read "VAR总磷总氮全局变量.vi" "状态告警区"() -> (w592:T4)
                  n316 = Unbundle By Name(w592) -> ("F0"=w589:sgl, "F1"=w588:sgl, "F2"=w587:sgl, "F3"=w586:sgl, "id"=w585:u16, "flowid"=w584:u16, "量程"=w583:u16)
                  n317 = Unbundle By Name(w595) -> ("id"=w573:u16)
                  n318 = call "id参数转换.vi"("id"=w573) -> ("table输出"=w572:string)  [unwired: 9 in, 1 out]
                  n319 = Concatenate Strings(w574, w578) -> (w575:string)
                  n320 = Format Into String(format string="F0=%#f,F1=%#f,F2=%#f,F3=%#f,Flow=%d-%-d-%-d" ("格式字符串"), w589, w588, w587, w586, w585, w584, w583) -> (resulting string=w590:string)  [unwired: 2 in, 1 out]
                  n321 = Get Date/Time In Seconds() -> (seconds since 1Jan1904=w593:timestamp)
                  n322 = Bundle By Name(cluster=T15 {"时间标识"=timestamp(0 s since 1904-01-01), "设备"="", "日志信息"="", "流程参数"=""} ("data in"), "时间标识"=w593, "设备"=w572, "日志信息"=w575, "流程参数"=w590) -> (w594:T15)
                  n323 = call "总磷总氮操作日志.vi"("data in"=w594) -> ()  [unwired: 10 in, 1 out]
                }
              }
            }
            n324 = local write "数组"(w551) -> ()
          }
          frame -1 {
          }
        }
      }
    }
    n325 = Not Equal?(x=w469, y=w497) -> (x != y?=w496:bool)
    n326 = Multiply(x=w475, y=100.0) -> (x*y=w472:dbl)
    "滑动杆" <- w472
    n327 = case shown="True" w496 {
      tunnel: w469 -> [_ w617]
      frame False {
      }
      frame True {
        n328 = Subtract(x=w617, y=1) -> (x-y=w615:i32)
        n329 = Subtract(x=w615, y=5) -> (x-y=w619:i32)
        n330 = Greater Or Equal To 0?(x=w619) -> (x >= 0?=w618:bool)
        n331 = property on="多列列表框" class="MCListbox (strict)"() -> (error out=w623:errorcluster, "TopLeft"=w624:T16)  [unwired: 2 in, 1 out]
        n332 = Select(t=w619, s=w618, f=0) -> (s? t:f=w620:i32)
        n333 = Bundle By Name(cluster=w624, "Row"=w620) -> (w625:T16)
        n334 = property on="多列列表框" class="MCListbox (strict)"(error in=w623, "TopLeft"=w625) -> ()  [unwired: 1 in, 2 out]
      }
    }
    n335 = global write "VAR总磷总氮全局变量.vi" "测试进度"(w472) -> ()
  }
  n336 = case shown="\"Idle\"" w14 {
    tunnel: w13 -> [w626 w630]
    tunnel: [w626 w627] -> w12
    frame "Bad", Default {
    }
    frame "Idle" {
      n337 = invoke class="VI" method="Run VI"(reference=w630, "Wait until done"=FALSE ("结束前等待"), "Auto Dispose Ref"=TRUE ("自动销毁引用")) -> (reference out=w627:refnum<vi>)  [unwired: 2 in, 4 out]
    }
  }
  n338 = case shown="\"Idle\"" w18 {
    tunnel: w17 -> [w631 w635]
    tunnel: [w631 w632] -> w16
    frame "Bad", Default {
    }
    frame "Idle" {
      n339 = invoke class="VI" method="Run VI"(reference=w635, "Wait until done"=FALSE ("结束前等待"), "Auto Dispose Ref"=TRUE ("自动销毁引用")) -> (reference out=w632:refnum<vi>)  [unwired: 2 in, 4 out]
    }
  }
  n340 = Obtain Notifier(name (unnamed)=w20, notification data type=FALSE) -> (notifier out=w21:refnum<notifier>)  [unwired: 2 in, 2 out]
  n341 = Obtain Queue(name (unnamed)=w20, element data type=cluster{"命令":string, "data":variant} {"命令"="", "data"=variant}) -> (queue out=w23:refnum<queue>)  [unwired: 3 in, 2 out]
  n342 = while {
    tunnel: w23 -> [w639]
    tunnel: w21 -> [w638]
    tunnel: w16 -> [w637]
    tunnel: w12 -> [w636]
    stop <- FALSE stop-if-true
    n343 = event shown="[10] \"停止\": Value Change" {
      selector: _ -> [_ _ _ _ _ _ _ _ _ _ _ _ _ _]
      dyn-events: _ -> [_ _ _ _ _ _ _ _ _ _ _ _ _ _]
      timeout: _ -> [_ _ _ _ _ _ _ _ _ _ _ _ _ _]
      tunnel: w639 -> [_ _ _ _ _ _ _ _ w653 _ w660 _ _ _]
      tunnel: w638 -> [_ _ _ _ _ _ _ _ _ _ w659 _ _ _]
      tunnel: w637 -> [_ _ _ _ _ _ _ _ _ _ _ w680 _ _]
      tunnel: w636 -> [_ _ _ _ _ _ _ _ _ _ _ _ w686 _]
      event Timeout {
        n344 = event-data() -> ()  [unwired: 1 in, 3 out]
      }
      event "流程操作": Value Change {
        n345 = event-data() -> ()  [unwired: 1 in, 6 out]
        n346 = global read "总磷总氮断电保存全局变量.vi" "简易流程路径"() -> (w641:path)
        n347 = global read "总磷总氮断电保存全局变量.vi" "流程路径"() -> (w642:path)
        n348 = call "流程批量写入.vi"("简易流程路径"=w641, "添加的路径"=w642) -> ()  [unwired: 10 in]
      }
      event "温度曲线": Value Change {
        n349 = event-data() -> ()  [unwired: 1 in, 6 out]
        n350 = call "温度曲线显示.vi"() -> ()  [unwired: 12 in]
      }
      event "试剂余量": Value Change {
        n351 = event-data() -> ()  [unwired: 1 in, 6 out]
        n352 = call "试剂余量显示UI.vi"() -> ()  [unwired: 12 in]
      }
      event "灯值调整": Value Change {
        n353 = event-data() -> ()  [unwired: 1 in, 6 out]
        n354 = call "灯值调整对话框.vi"() -> ()  [unwired: 12 in]
      }
      event "布尔": Value Change {
        n355 = event-data() -> ("NewVal"=w643:bool)  [unwired: 1 in, 5 out]
        n356 = case shown="False" w643 {
          frame False {
            n357 = global write "VAR总磷总氮全局变量.vi" "权限等级"(enum16{"一级权限", "二级权限", "三级权限", "超级权限"}."一级权限" ("权限等级")) -> ()
          }
          frame True {
            n358 = global read "VAR总磷总氮全局变量.vi" "权限密码"() -> (w647:u32[])
            n359 = global read "VAR总磷总氮全局变量.vi" "权限等级"() -> (w645:enum16{"一级权限", "二级权限", "三级权限", "超级权限"})
            n360 = call "密码权限设置.vi"("权限输入"=w645, "权限密码"=w647) -> ("权限输出"=w646:enum16{"一级权限", "二级权限", "三级权限", "超级权限"})  [unwired: 9 in]
            n361 = global write "VAR总磷总氮全局变量.vi" "权限等级"(w646) -> ()
          }
        }
      }
      event "权限等级": Mouse Down {
        n362 = event-data() -> ()  [unwired: 1 in, 8 out]
        n363 = global read "VAR总磷总氮全局变量.vi" "权限密码"() -> (w650:u32[])
        n364 = global read "VAR总磷总氮全局变量.vi" "权限等级"() -> (w648:enum16{"一级权限", "二级权限", "三级权限", "超级权限"})
        n365 = call "密码权限设置.vi"("权限输入"=w648, "权限密码"=w650) -> ("权限输出"=w649:enum16{"一级权限", "二级权限", "三级权限", "超级权限"})  [unwired: 9 in]
        n366 = global write "VAR总磷总氮全局变量.vi" "权限等级"(w649) -> ()
      }
      event "外设固件": Value Change {
        n367 = event-data() -> ()  [unwired: 1 in, 6 out]
        n368 = call "流程固件设置对话框.vi"() -> ()  [unwired: 12 in]
      }
      event "手动启动": Value Change {
        n369 = event-data() -> ()  [unwired: 1 in, 6 out]
        n370 = call "总磷总氮启动参数对话框.vi"() -> ("确认"=w651:bool, "元素"=w652:cluster{"命令":string, "data":variant})  [unwired: 10 in]
        n371 = case shown="True" w651 {
          tunnel: w653 -> [_ w656]
          tunnel: w652 -> [_ w655]
          frame False {
          }
          frame True {
            n372 = Flush Queue(queue=w656) -> (queue out=w654:refnum<queue>)  [unwired: 1 in, 2 out]
            n373 = Enqueue Element(queue=w654, element=w655) -> ()  [unwired: 2 in, 3 out]
          }
        }
      }
      event "调试": Value Change {
        n374 = event-data() -> ()  [unwired: 1 in, 6 out]
        n375 = call "简易流程调试界面.vi"() -> ()  [unwired: 12 in]
      }
      event "停止": Value Change {
        n376 = event-data() -> ()  [unwired: 1 in, 6 out]
        n377 = Two Button Dialog(message="确认停止？" ("消息")) -> (T button?=w657:bool)  [unwired: 2 in]
        n378 = case shown="True" w657 {
          tunnel: w660 -> [_ w676]
          tunnel: w659 -> [_ w675]
          frame False {
          }
          frame True {
            n379 = Send Notification(notification=TRUE ("通知"), notifier=w675) -> ()  [unwired: 1 in, 2 out]
            n380 = global read "VAR总磷总氮全局变量.vi" "状态告警区"() -> (w670:T4)
            n381 = global read "VAR总磷总氮全局变量.vi" "状态告警区"() -> (w662:T4)
            n382 = Unbundle By Name(w670) -> ("id"=w669:u16)
            n383 = Unbundle By Name(w662) -> ("id"=w661:u16)
            n384 = Bundle By Name(cluster=T18 {"站号"=1, "量程切换"=enum."AUTO", "控制命令"=enum."停止测试", "模式设置"=enum."待机", "测量间隔"=0} ("参数"), "站号"=w669) -> (w671:T18)
            n385 = call "id参数转换.vi"("id"=w661) -> ("table输出"=w663:string)  [unwired: 9 in, 1 out]
            n386 = call "总磷总氮启动命令.vi"("参数"=w671) -> ("启动命令"=w672:cluster{"命令":string, "data":variant})  [unwired: 10 in]
            n387 = Get Date/Time In Seconds() -> (seconds since 1Jan1904=w666:timestamp)
            n388 = Bundle By Name(cluster=T17 {"时间"=timestamp(0 s since 1904-01-01), "参数"="", "日志信息"="", "流程参数"=""} ("data in"), "时间"=w666, "参数"=w663, "日志信息"="手动停止") -> (w667:T17)
            n389 = Enqueue Element(queue=w676, element=w672) -> (error out=w664:errorcluster)  [unwired: 2 in, 2 out]
            n390 = call "总磷总氮操作日志.vi"("错误输入（无错误）"=w664, "data in"=w667) -> ()  [unwired: 9 in, 1 out]
          }
        }
      }
      event "参数设置", "参数查询": Value Change {
        n391 = event-data() -> ()  [unwired: 1 in, 6 out]
        n392 = invoke on="子面板" class="SubPnl" method="Remove VI"() -> (error out=w681:errorcluster)  [unwired: 3 in, 2 out]
        n393 = property on="仪器校准" class="Bool"("Visible"=TRUE ("可见")) -> ()  [unwired: 2 in, 2 out]
        n394 = property on="参数查询" class="Bool"("Visible"=FALSE ("可见")) -> ()  [unwired: 2 in, 2 out]
        n395 = property on="窗格" class="Pane"("Origin"=T3 {"Horizontal"=0, "Vertical"=640} ("原点")) -> ()  [unwired: 2 in, 2 out]
        n396 = invoke on="子面板" class="SubPnl" method="Insert VI"(error in=w681, "VI Ref"=w680) -> ()  [unwired: 2 in, 4 out]
        n397 = global write "VAR总磷总氮全局变量.vi" "页面"(enum16{"主页", "参数页", "校准页"}."参数页" ("页面")) -> ()
      }
      event "仪器校准": Value Change {
        n398 = event-data() -> ()  [unwired: 1 in, 6 out]
        n399 = invoke on="子面板" class="SubPnl" method="Remove VI"() -> (error out=w687:errorcluster)  [unwired: 3 in, 2 out]
        n400 = property on="仪器校准" class="Bool"("Visible"=FALSE ("可见")) -> ()  [unwired: 2 in, 2 out]
        n401 = property on="参数查询" class="Bool"("Visible"=TRUE ("可见")) -> ()  [unwired: 2 in, 2 out]
        n402 = global write "VAR总磷总氮全局变量.vi" "页面"(enum16{"主页", "参数页", "校准页"}."校准页" ("页面")) -> ()
        n403 = invoke on="子面板" class="SubPnl" method="Insert VI"(error in=w687, "VI Ref"=w686) -> ()  [unwired: 2 in, 4 out]
      }
      event "返回": Value Change {
        n404 = event-data() -> ()  [unwired: 1 in, 6 out]
        n405 = global write "VAR总磷总氮全局变量.vi" "页面"(enum16{"主页", "参数页", "校准页"}."主页" ("页面")) -> ()
        n406 = property on="窗格" class="Pane"("Origin"=T3 {"Horizontal"=0, "Vertical"=0} ("原点")) -> ()  [unwired: 2 in, 2 out]
      }
    }
  }
  n407 = while {
    tunnel: w23 -> [w701]
    stop <- FALSE stop-if-true
    n408 = Wait (ms)(milliseconds to wait=u32 1000 ("等待时间（毫秒）")) -> ()  [unwired: 1 out]
    n409 = global read "总磷总氮断电保存全局变量.vi" "MB通信方式选择"() -> (w699:enum16{"串口", "TCP"})
    n410 = global read "VAR总磷总氮全局变量.vi" "升级固件关闭心跳包"() -> (w693:bool)
    n411 = global read "VAR总磷总氮全局变量.vi" "MB session in"() -> (w697:refnum<class "MB_Master.lvclass">)
    n412 = case shown="\"串口\", Default" w699 {
      tunnel: [w704 w705] -> w698
      frame "串口", Default {
        n413 = global read "总磷总氮断电保存全局变量.vi" "VISA Resource"() -> (w704:refnum<visa-resource-name>)
      }
      frame "TCP" {
        n414 = global read "总磷总氮断电保存全局变量.vi" "IP"() -> (w705:string)
      }
    }
    "字符串 2" <- w698
    n415 = property class="MB_Master"(reference=w697) -> ("Properties:Session Valid"=w695:bool)  [unwired: 1 in, 2 out]
    n416 = Not(x=w693) -> (.not. x?=w692:bool)
    n417 = Get Queue Status(queue=w701) -> (queue out=w700:refnum<queue>, # elements in queue=w696:i32)  [unwired: 2 in, 6 out]
    n418 = Equal To 0?(x=w696) -> (x = 0?=w690:bool)
    n419 = Compound Arithmetic op=AND ("复合运算")(w695, w692) -> (w694:bool)
    n420 = global write "VAR总磷总氮全局变量.vi" "心跳包打开状态"(w694) -> ()
    n421 = And(x=w690, y=w694) -> (x .and. y?=w691:bool)
    n422 = case shown="True" w691 {
      tunnel: w700 -> [_ w724]
      frame False {
      }
      frame True {
        n423 = global read "VAR总磷总氮全局变量.vi" "MB session in"() -> (w712:refnum<class "MB_Master.lvclass">)
        n424 = property class="MB_Master"(reference=w712) -> ("Properties:Session Valid"=w710:bool)  [unwired: 1 in, 2 out]
        n425 = global read "VAR总磷总氮全局变量.vi" "通讯状态"() -> (w713:bool)
        n426 = case shown="True" w710 {
          tunnel: [_ w726] -> w709
          frame False {
          }
          frame True {
            n427 = global read "VAR总磷总氮全局变量.vi" "MB session in"() -> (w725:refnum<class "MB_Master.lvclass">)
            n428 = call "版本号读取.vi"("MB session in"=w725) -> ("error out"=w726:errorcluster, "固件版本号"=w727:string)  [unwired: 8 in, 1 out]
            "固件版本号" <- w727
            n429 = global write "VAR总磷总氮全局变量.vi" "固件版本号"(w727) -> ()
          }
        }
        n430 = And(x=w710, y=w713) -> (x .and. y?=w711:bool)
        n431 = case shown="True" w711 {
          tunnel: [_ w728] -> w708
          tunnel: w709 -> [_ w729]
          frame False {
          }
          frame True {
            n432 = global read "VAR总磷总氮全局变量.vi" "MB session in"() -> (w731:refnum<class "MB_Master.lvclass">)
            n433 = call "序列号读取.vi"("Error in"=w729, "MB session in"=w731) -> ("error out"=w728:errorcluster, "序列号"=w730:string)  [unwired: 7 in, 1 out]
            n434 = global write "VAR总磷总氮全局变量.vi" "序列号"(w730) -> ()
          }
        }
        n435 = global read "model config var.vi" "启动队列名称"() -> (w715:cluster{"String":string, "Value":u16}[])
        n436 = for {
          tunnel: [w742] -> w716 mode=indexing
          tunnel: w715 -> [w743] mode=indexing
          tunnel: w708 -> [_]
          n437 = Unbundle By Name(w743) -> ("Value"=w742:u16)
        }
        n438 = for {
          shift-right: [w732] -> w718
          shift-left: w724 -> [w738]
          tunnel: w716 -> [w733] mode=indexing
          n439 = Bundle By Name(cluster=cluster{"命令":string, "data":variant} {"命令"="", "data"=variant} ("元素"), "命令"="读状态告警区", "data"=w733) -> (w740:cluster{"命令":string, "data":variant})
          n440 = Bundle By Name(cluster=cluster{"命令":string, "data":variant} {"命令"="", "data"=variant} ("元素"), "命令"="读测量数据区", "data"=w733) -> (w735:cluster{"命令":string, "data":variant})
          n441 = Enqueue Element(queue=w738, element=w740) -> (queue out=w734:refnum<queue>)  [unwired: 2 in, 2 out]
          n442 = Enqueue Element At Opposite End(queue=w734, element=w735) -> (queue out=w732:refnum<queue>)  [unwired: 2 in, 2 out]
        }
        n443 = global read "VAR总磷总氮全局变量.vi" "状态告警区"() -> (w717:T4)
        n444 = Unbundle By Name(w717) -> ("系统时间"=w706:timestamp)
        n445 = Get Date/Time In Seconds() -> (seconds since 1Jan1904=w723:timestamp)
        n446 = Subtract(x=w723, y=w706) -> (x-y=w722:dbl)
        n447 = Absolute Value(x=w722) -> (abs(x)=w721:dbl)
        n448 = global read "VAR总磷总氮全局变量.vi" "通讯状态"() -> (w707:bool)
        n449 = Greater Or Equal?(x=w721, y=30.0) -> (x >= y?=w719:bool)
        n450 = Compound Arithmetic op=AND ("复合运算")(w719, w707) -> (w714:bool)
        n451 = case shown="True" w714 {
          tunnel: w718 -> [_ w745]
          frame False {
          }
          frame True {
            n452 = call "总磷总氮启动命令.vi"("参数"=T18 {"站号"=3, "量程切换"=enum."AUTO", "控制命令"=enum."校时", "模式设置"=enum."待机", "测量间隔"=0}) -> ("启动命令"=w744:cluster{"命令":string, "data":variant})  [unwired: 10 in]
            n453 = Enqueue Element(queue=w745, element=w744) -> ()  [unwired: 2 in, 3 out]
          }
        }
      }
    }
  }
